vi "Get Status (SubVI).vi"(5 "Image Height":u16, 7 "Image Width":u16, 8 "Input Valid?":bool, 11 "Pixel In":u64) -> (0 "Pixel Valid?":bool, 3 "Pixel Out":u64, 4 "Frame Interval":u32=4294967295, 6 "Frame #":u32)   [LabVIEW 2015]
uses:
  <vilib>/rvi/interface/RandomDataEmulation/niFpgaRandomDataHandleErrors.vi
  <vilib>/rvi/DataTransferAndStorage/Container/XNode/niFpgaContainer.xnode
  <vilib>/rvi/interface/RandomDataEmulation/nirviRandomDataFpgaReadWriteTemplate.vi
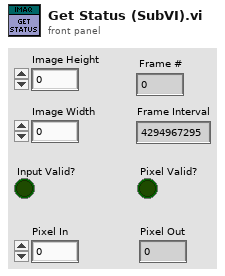
[diagram p1: front panel]
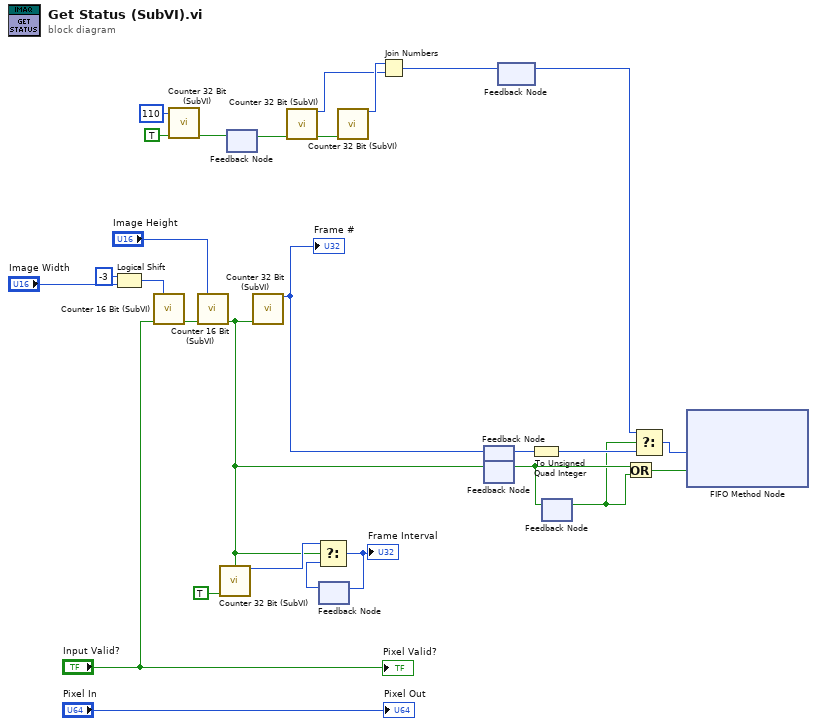
[diagram p0: block diagram]
diagram:
  n1 = Logical Shift(y=i16 -3, x="Image Width") -> (x << y=w21:u16)
  n2 = call "Counter 16 Bit (SubVI).vi"("Max. Count"=w21, "Enable"="Input Valid?") -> ("Count End?"=w22:bool)  [unwired: 11 in, 2 out]
  n3 = call "Counter 32 Bit (SubVI).vi"("Max. Count"=u32 110, "Enable"=TRUE) -> ("Count End?"=w16:bool)  [unwired: 11 in, 2 out]
  n4 = call "Counter 16 Bit (SubVI).vi"("Max. Count"="Image Height", "Enable"=w22) -> ("Count End?"=w10:bool)  [unwired: 11 in, 2 out]
  n5 = call "Counter 32 Bit (SubVI).vi"("RESET"=w10, "Enable"=TRUE) -> ("Count"=w24:u32)  [unwired: 11 in, 2 out]
  n6 = feedback-in #1(w16) -> ()
  n7 = feedback #1() -> (w15:bool)  [unwired: 1 in]
  n8 = call "Counter 32 Bit (SubVI).vi"("Enable"=w10) -> ("Count"=w9:u32)  [unwired: 12 in, 2 out]
  "Frame #" <- w9
  n9 = call "Counter 32 Bit (SubVI).vi"("Enable"=w15) -> ("Count"=w12:u32, "Count End?"=w14:bool)  [unwired: 12 in, 1 out]
  n10 = feedback #2() -> (w25:u32)  [unwired: 1 in]
  n11 = Select(t=w24, s=w10, f=w25) -> (s? t:f=w26:u32)
  "Frame Interval" <- w26
  n12 = feedback-in #2(w26) -> ()
  n13 = call "Counter 32 Bit (SubVI).vi"("Enable"=w14) -> ("Count"=w13:u32)  [unwired: 12 in, 2 out]
  n14 = Join Numbers(hi=w13, lo=w12) -> ((hi.lo)=w2:u64)
  n15 = feedback-in #3(w9) -> ()
  n16 = feedback #3() -> (w8:u32)  [unwired: 1 in]
  n17 = feedback-in #4(w10) -> ()
  n18 = feedback #4() -> (w6:bool)  [unwired: 1 in]
  n19 = feedback-in #5(w2) -> ()
  n20 = feedback #5() -> (w1:u64)  [unwired: 1 in]
  n21 = To Unsigned Quad Integer(1:w8) -> (0:w7:u64)
  n22 = feedback #6() -> (w3:bool)  [unwired: 1 in]
  n23 = feedback-in #6(w6) -> ()
  n24 = Or(x=w6, y=w3) -> (x .or. y?=w5:bool)
  n25 = Select(t=w1, s=w3, f=w7) -> (s? t:f=w4:u64)
  n26 = xnode ("FIFO Method Node")("Element"=w4, "Input Valid"=w5) -> ()  [unwired: 1 in, 2 out]
  "Pixel Out" <- "Pixel In"
  "Pixel Valid?" <- "Input Valid?"
